vi "Delete and Copy Template.vi"(9 "Code Template":string, 10 "Code Root":string, 11 "Project Root":path) -> ()   [LabVIEW 2020]
panel:
  # "SubVI\nDo Not Run Directly"
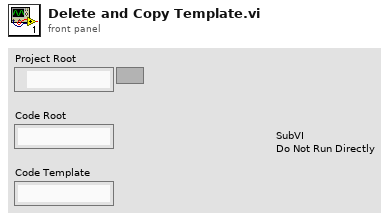
[diagram p1: front panel]
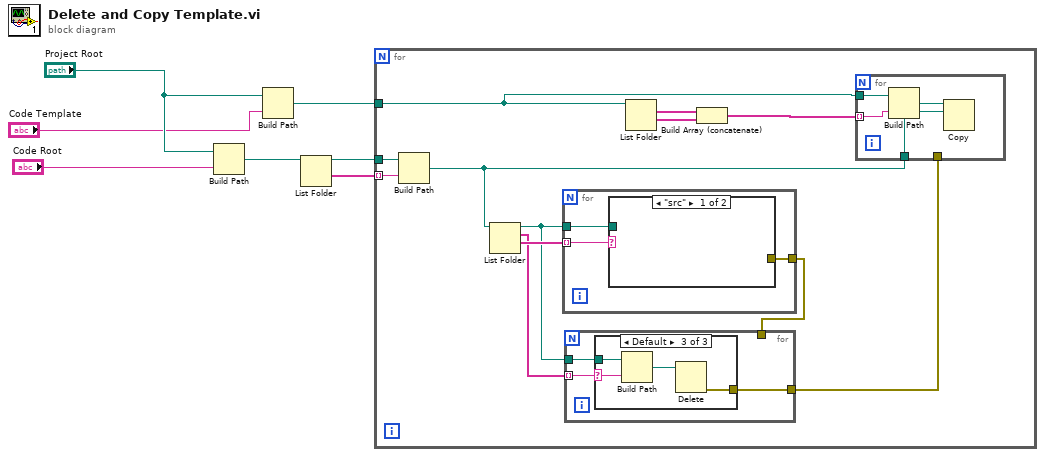
[diagram p0: block diagram]
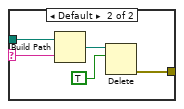
[diagram p4: hidden frame]
diagram:
  n1 = Build Path(base path="Project Root", name or relative path="Code Root") -> (appended path=w3:path)
  n2 = Build Path(base path="Project Root", name or relative path="Code Template") -> (appended path=w7:path)
  n3 = List Folder(path=w3) -> (path out=w6:path, folder names=w2:string[])  [unwired: 3 in, 2 out]
  n4 = for {
    tunnel: w2 -> [w19] mode=indexing
    tunnel: w6 -> [w18]
    tunnel: w7 -> [w10]
    n5 = Build Path(base path=w18, name or relative path=w19) -> (appended path=w13:path)
    n6 = List Folder(path=w13) -> (path out=w15:path, filenames=w16:string[], folder names=w17:string[])  [unwired: 3 in, 1 out]
    n7 = for {
      tunnel: w17 -> [w32] mode=indexing
      tunnel: w15 -> [w33]
      tunnel: [w31] -> w14
      n8 = case shown="\"src\"" w32 {
        selector: w32 -> [_ w37]
        tunnel: w33 -> [_ w38]
        tunnel: [_ w34] -> w31
        frame "src" {
        }
        frame Default {
          n9 = Build Path(base path=w38, name or relative path=w37) -> (appended path=w36:path)
          n10 = Delete(path (use dialog)=w36, entire hierarchy (F)=TRUE) -> (error out=w34:errorcluster)  [unwired: 3 in, 2 out]
        }
      }
    }
    n11 = for {
      tunnel: w16 -> [w24] mode=indexing
      tunnel: w15 -> [w26]
      tunnel: [w25] -> w8
      tunnel: w14 -> [_]
      n12 = case shown="Default" w24 {
        selector: w24 -> [_ _ w27]
        tunnel: w26 -> [_ _ w30]
        tunnel: [_ _ w28] -> w25
        frame "README.md" {
        }
        frame "shuffleboard.json" {
        }
        frame Default {
          n13 = Build Path(base path=w30, name or relative path=w27) -> (appended path=w29:path)
          n14 = Delete(path (use dialog)=w29) -> (error out=w28:errorcluster)  [unwired: 4 in, 2 out]
        }
      }
    }
    n15 = List Folder(path=w10) -> (filenames=w11:string[], folder names=w12:string[])  [unwired: 3 in, 2 out]
    n16 = Build Array (concatenate)(w11, w12) -> (w9:string[])
    n17 = for {
      tunnel: w13 -> [w23]
      tunnel: w10 -> [w22]
      tunnel: w9 -> [w21] mode=indexing
      tunnel: w8 -> [_]
      n18 = Build Path(base path=w22, name or relative path=w21) -> (appended path=w20:path)
      n19 = Copy(10:w23, 11:w20) -> ()  [unwired: 3 in, 3 out]
    }
  }
